vi "Top Filled Slot.vi"(11 "Room":string[](array[string])) -> (3 "Top Filled Slot":i32)   [LabVIEW 2019, in "23.lvlib"]
uses:
  23.lvlib
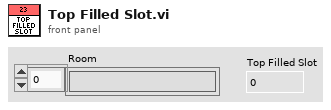
[diagram p1: front panel]
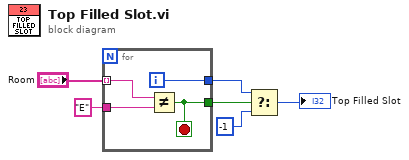
[diagram p0: block diagram]
diagram:
  n1 = for {
    tunnel: "Room" -> [w10] mode=indexing
    tunnel: "E" ("y") -> [w9]
    tunnel: [w8] -> w2
    tunnel: [w7] -> w3
    i -> [w8]
    stop <- w7 stop-if-true
    n2 = Not Equal?(x=w10, y=w9) -> (x != y?=w7:bool)
  }
  n3 = Select(t=w2, s=w3, f=-1) -> (s? t:f=→"Top Filled Slot":i32)
